vi "Validate.vi"(8 "error in":errorcluster, 10 "Obj Dictionary":refnum<class "Object Dictionary.lvclass">, 11 "CiA401 Generic IO Profile in":refnum<class "CiA401 Generic IO Profile.lvclass">) -> (0 "error out":errorcluster, 2 "Validation Messages":T1[](array[typedef]) {"Sub Index" format="%02x"; "Index" format="%04x"}, 3 "CiA401 Generic IO Profile out":refnum<class "CiA401 Generic IO Profile.lvclass">)   [LabVIEW 2020, in "CiA401 Generic IO Profile.lvclass"]
uses:
  CiA401 Generic IO Profile.lvclass
  CiA401 Generic IO Profile.lvclass/CiA401 Generic IO Profile.ctl
  source/Object Dictionary/Object Dictionary.lvclass
  source/Typedefs/Validation Severity.ctl
  source/CANopen.lvlib
  source/Typedefs/Validation Message.ctl
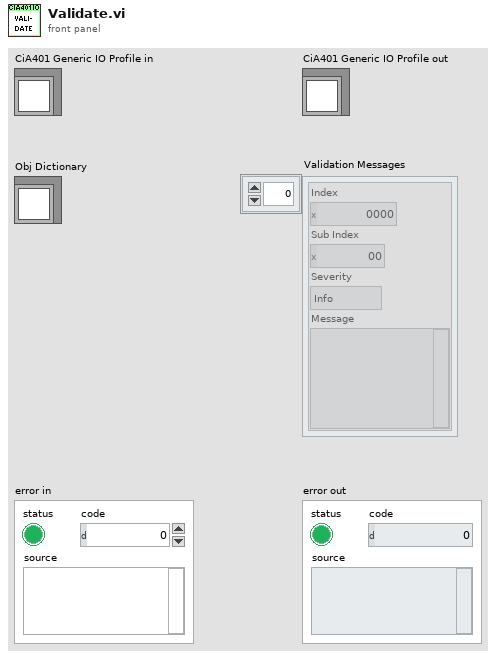
[diagram p1: front panel]
types:
  T1 = typedef "CANopen.lvlib/Validation Message.ctl" = cluster{"Index":u16, "Sub Index":u8, "Severity":T2, "Message":string}
  T2 = typedef "CANopen.lvlib/Validation Severity.ctl" = enum16{"Info", "Warning", "Error"}
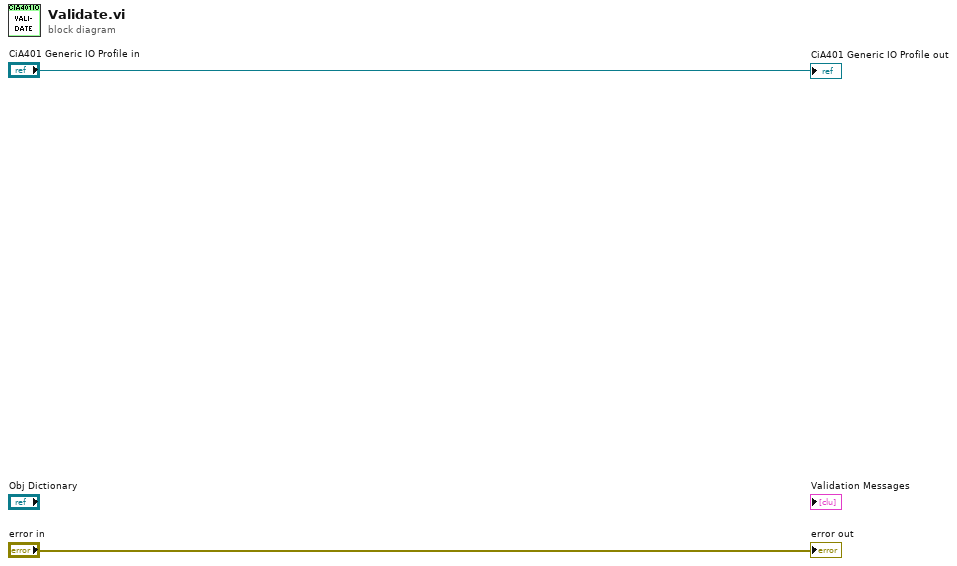
[diagram p0: block diagram]
diagram:
  "CiA401 Generic IO Profile out" <- "CiA401 Generic IO Profile in"
  "error out" <- "error in"
